vi "4_Main.vi"() -> ()   [LabVIEW 2015, in "TestActor.lvlib"]
doc: "This is the main VI for the exercise in chapter 4."
uses:
  TestActor/TestActor.lvlib
  TestActor/TestActor.lvclass
  CSPP_Core/Classes/CS++BaseClasses/Factory/CS++Factory.lvclass
  CSPP_Core/Classes/CS++BaseClasses/Factory/CS++Factory.lvclass/CS++Factory.ctl
  <vilib>/ActorFramework/Message Enqueuer/Message Enqueuer.lvclass/Message Enqueuer.ctl
  <vilib>/ActorFramework/Message Enqueuer/Enqueue.vi
  <vilib>/ActorFramework/Message Priority Queue/Priority Enqueue.vi
  TestActor Messages/Zero Msg/Zero Msg.lvclass
  <vilib>/ActorFramework/Stop Msg/Stop Msg.lvclass
  <vilib>/ActorFramework/Actor/Actor.lvclass
  CSPP_Core/Classes/CS++ProcessVariables/CS++ProcessVariables.lvlib
panel:
  in  "Zero":bool
  in  "Stop":bool
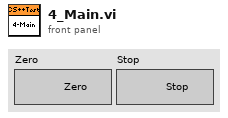
[diagram p1: front panel]
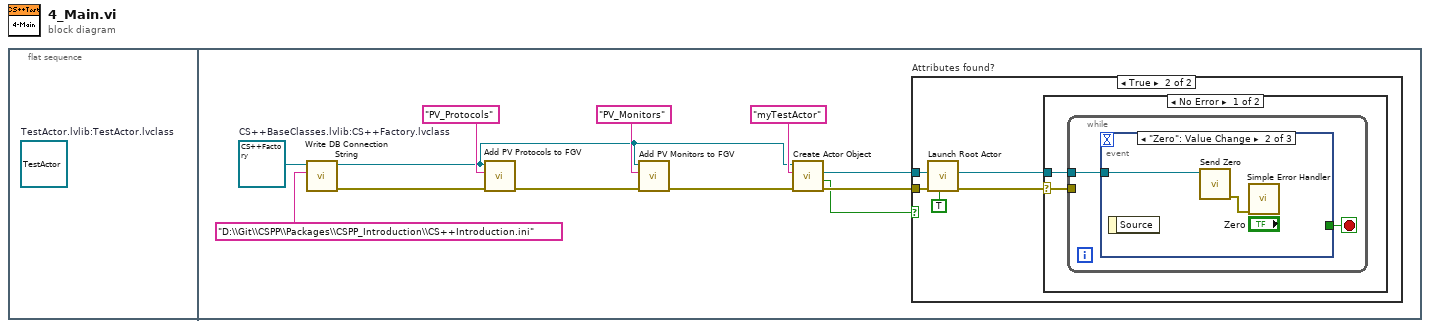
[diagram p0: block diagram]
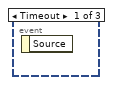
[diagram p3: hidden frame]
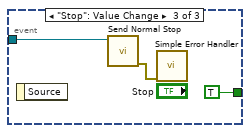
[diagram p4: hidden frame]
diagram:
  n1 = flat-sequence {
    frame #0 {
      (unwired) refnum<class "TestActor.lvclass"> refnum  # TestActor.lvlib:TestActor.lvclass
    }
    frame #1 {
      w12 = refnum<class "CS++Factory.lvclass"> refnum  # CS++BaseClasses.lvlib:CS++Factory.lvclass
      n2 = call "Write DB Connection String.vi"("DB Connection String"="D:\\Git\\CSPP\\Packages\\CSPP_Introduction\\CS++Introduction.ini", "CS++Factory in"=w12) -> ("error out"=w3:errorcluster, "CS++Factory out"=w1:refnum<class "CS++Factory.lvclass">)  [unwired: 8 in]
      n3 = call "Add PV Protocols to FGV.vi"("Error In"=w3, "PV Protocol Section"="PV_Protocols" ("string"), "CS++Factory"=w1) -> ("Error Out"=w6:errorcluster)  [unwired: 8 in]
      n4 = call "Add PV Monitors to FGV.vi"("Error In"=w6, "PV Monitor Section"="PV_Monitors", "CS++Factory"=w1) -> ("Error Out"=w2:errorcluster)  [unwired: 8 in]
      n5 = call "Create Actor Object.vi"("error in (no error)"=w2, "Object Name"="myTestActor", "CS++Factory in"=w1) -> ("error out"=w10:errorcluster, "Attributes found?"=w9:bool, "CS++BaseActor"=w11:refnum<class "CS++BaseActor.lvclass">)  [unwired: 5 in, 1 out]
      n6 = case "Attributes found?" shown="True" w9 {
        tunnel: w11 -> [_ w14]
        tunnel: w10 -> [_ w17]
        frame False {
        }
        frame True {
          n7 = call <vilib>:"Launch Root Actor.vi"("Open Actor Core front panel? (F)"=TRUE, "error in (no error)"=w17, "Actor"=w14) -> ("error out"=w16:errorcluster, "Actor's Enqueuer"=w15:refnum<class "Message Enqueuer.lvclass">)  [unwired: 7 in]
          n8 = case shown="No Error" w16 {
            selector: w16 -> [w19 _]
            tunnel: w15 -> [w18 _]
            frame No Error {
              n9 = while {
                tunnel: w19 -> [_]
                tunnel: w18 -> [w21]
                stop <- w20 stop-if-true
                n10 = event shown="[1] \"Zero\": Value Change" {
                  selector: _ -> [_ _ _]
                  dyn-events: _ -> [_ _ _]
                  timeout: _ -> [_ _ _]
                  tunnel: w21 -> [_ w23 w26]
                  tunnel: [_ _ TRUE] -> w20
                  event Timeout {
                    n11 = event-data() -> ()  [unwired: 1 in, 1 out]
                  }
                  event "Zero": Value Change {
                    n12 = event-data() -> ()  [unwired: 1 in, 1 out]
                    n13 = call "Send Zero.vi"("Message Enqueuer"=w23) -> ("error out"=w22:errorcluster)  [unwired: 9 in, 1 out]
                    n14 = call <vilib>:"Simple Error Handler.vi"("error in (no error)"=w22) -> ()  [unwired: 4 in, 5 out]
                  }
                  event "Stop": Value Change {
                    n15 = event-data() -> ()  [unwired: 1 in, 1 out]
                    n16 = call <vilib>:"Send Normal Stop.vi"("Message Enqueuer"=w26) -> ("error out"=w25:errorcluster)  [unwired: 10 in]
                    n17 = call <vilib>:"Simple Error Handler.vi"("error in (no error)"=w25) -> ()  [unwired: 4 in, 5 out]
                  }
                }
              }
            }
            frame Error {
            }
          }
        }
      }
    }
  }
